vi "Lockin.Create Notch Filter (FGV).vi"(6 "fs (Hz)":dbl, 7 "init [F]":bool, 8 "error in (no error)":errorcluster) -> (0 "error out":errorcluster, 2 "filters out":T1[](array[typedef]) {"mSRate_QSettings"."source" items=["Coef a/k"=0, "Coef b/v"=7, "Input"=1, "Output"=2, "Multiplicand"=3, "Product"=4, "Sum"=5, "Delay"=6, "Gain"=8]}, 5 "init?":bool)   [LabVIEW 2019, in "DSP.lvclass"]
uses:
  DSP.lvclass
  <vilib>/addons/Digital Filter Design/_Objects.llb/DFD Filter Obj.ctl
  <vilib>/addons/Digital Filter Design/_Objects.llb/DFD Filter Coef.ctl
  <vilib>/addons/Digital Filter Design/_Objects.llb/DFD Filter Structure Type Selector.ctl
  <vilib>/addons/Digital Filter Design/_Objects.llb/dfd_Internal Quantization Settings.ctl
  <vilib>/addons/Digital Filter Design/_Objects.llb/dfd_Internal Quantization Srcs.ctl
  <vilib>/addons/Digital Filter Design/_Objects.llb/DFD Coef Norm Type.ctl
  <vilib>/addons/Digital Filter Design/Design.llb/DFD IIR Notch Peak Design by Q.vi
  <vilib>/addons/Digital Filter Design/NI_DigFilterLicensed.lvlib
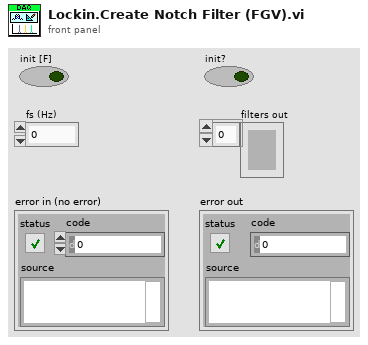
[diagram p1: front panel]
types:
  T1 = typedef "NI_DigFilterLicensed.lvlib/DFD Filter Obj.ctl" = cluster{"mSRate_Fs":dbl, "mSRate_Version":string, "mSRate_Comments":string, "mSRate_OrgCoef":T2, "mSRate_CurCoef":T2, "mSRate_Quantized?":bool, "mSRate_QCoef":T2, "mSRate_QSettings":T4[], "mSRate_Order":i32, "mSRate_Scaling":cluster{"mSRate_ScaleByPowerOf2?":bool, "mSRate_ScaleType":T6}}
  T2 = typedef "NI_DigFilterLicensed.lvlib/DFD Filter Coef.ctl" = cluster{"type":T3, "gain":dbl, "coef a (k)":dbl[], "coef b (v)":dbl[]}
  T3 = typedef "NI_DigFilterLicensed.lvlib/DFD Filter Structure Type Selector.ctl" = enum16{"Undefined", "FIR Direct Form", "FIR Direct Form Transposed", "FIR Symmetric", "FIR Antisymmetric", "IIR Direct Form I", "IIR Direct Form I Transposed", "IIR Direct Form II", "IIR Direct Form II Transposed", "IIR Cascaded Second Order Sections Form I", "IIR Cascaded Second Order Sections Form I Transposed", "IIR Cascaded Second Order Sections Form II", "IIR Cascaded Second Order Sections Form II Transposed", "Lattice Allpass (basic sections)", "Lattice Allpass (one multiplier sections)", "Lattice Allpass (normalized sections)", "Lattice AR (basic sections)", "Lattice AR (one multiplier sections)", "Lattice AR (normalized sections)", "Lattice MA (minimum phase)", "Lattice MA (maximum phase)", "Lattice ARMA (basic sections)", "Lattice ARMA (one multiplier sections)", "Lattice ARMA (normalized sections)"}
  T4 = typedef "NI_DigFilterLicensed.lvlib/dfd_Internal Quantization Settings.ctl" = cluster{"source":T5, "wl":i16, "iwl":i16, "overflow mode":enum16{"Saturation", "Wrap"}, "rounding mode":enum16{"Nearest", "Truncation"}, "signed?":bool}
  T5 = typedef "NI_DigFilterLicensed.lvlib/dfd_Internal Quantization Srcs.ctl" = u16
  T6 = typedef "NI_DigFilterLicensed.lvlib/DFD Coef Norm Type.ctl" = enum16{"No Norm", "Time Domain 1-Norm", "Time Domain 2-Norm", "Time Domain Inf-Norm"}
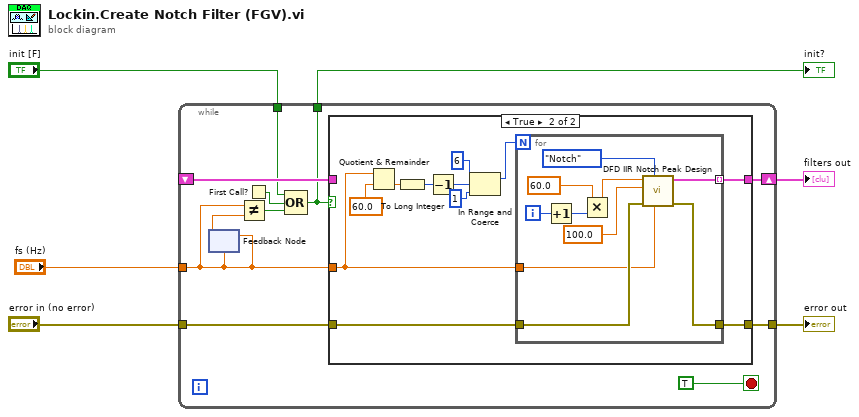
[diagram p0: block diagram]
diagram:
  n1 = while {
    shift-right: [w16] -> w5
    shift-left: _ -> [w9]
    tunnel: "fs (Hz)" -> [w15]
    tunnel: "error in (no error)" -> [w17]
    tunnel: [w10] -> w3
    tunnel: "init [F]" -> [w8]
    tunnel: [w7] -> w6
    stop <- TRUE stop-if-true
    n2 = feedback #1(w15) -> (w14:dbl)
    n3 = feedback-in #1(w15) -> ()
    n4 = Not Equal?(x=w15, y=w14) -> (x != y?=w13:bool)
    n5 = First Call?() -> (First Call?: T/F=w12:bool)
    n6 = Compound Arithmetic op=OR(w8, w12, w13) -> (w7:bool)
    n7 = case shown="True" w7 {
      tunnel: w17 -> [w18 w30]
      tunnel: [w19 w28] -> w16
      tunnel: w15 -> [_ w29]
      tunnel: [w18 w27] -> w10
      tunnel: w9 -> [w19 _]
      frame False {
      }
      frame True {
        n8 = Quotient & Remainder(x=w29, y=60.0 ("f0 [Hz]")) -> (floor(x/y)=w25:dbl)  [unwired: 1 out]
        n9 = To Long Integer(number=w25) -> (32bit integer=w26:i32)
        n10 = Decrement(x=w26) -> (x-1=w23:i32)
        n11 = In Range and Coerce(upper limit=6, x=w23, lower limit=1) -> (coerced(x)=w20:i32)  [unwired: 1 out]
        n12 = for {
          N: w20 -> [_]
          tunnel: w29 -> [w31]
          tunnel: [w32] -> w28 mode=indexing
          tunnel: w30 -> [w40]
          tunnel: [w33] -> w27
          i -> [w35]
          n13 = Increment(x=w35) -> (x+1=w37:i32)
          n14 = Multiply(x=60.0 ("f0 [Hz]"), y=w37) -> (x*y=w34:dbl)
          n15 = call-poly <vilib>:"DFD IIR Notch Peak Design.vi"("fs [Hz]"=w31, "filter type"=enum16{"Notch", "Peak"}."Notch", "error in (no error)"=w40, "Q factor"=100.0, "f0 [Hz]"=w34) -> ("error out"=w33:errorcluster, "filter out"=w32:T1)  [unwired: 5 in]
        }
      }
    }
  }
  "init?" <- w6
  "filters out" <- w5
  "error out" <- w3
